vi "PathPlanner_Waypoint_New.vi"(9 "NextControl":T1={"X"=-9.9e+30, "Y"=-9.9e+30} {"Y" format="%14.3f"; "X" format="%14.3f"}, 10 "Anchor":T1 {"Y" format="%14.3f"; "X" format="%14.3f"}, 11 "PrevControl":T1={"X"=-9.9e+30, "Y"=-9.9e+30} {"Y" format="%14.3f"; "X" format="%14.3f"}) -> (3 "Waypoint":T2 {"nextControl"."Y" format="%14.3f"; "nextControl"."X" format="%14.3f"; "anchor"."Y" format="%14.3f"; "anchor"."X" format="%14.3f"; "prevControl"."Y" format="%14.3f"; "prevControl"."X" format="%14.3f"})   [LabVIEW 2019, in "PathPlanner24.lvlib"]
doc: "Convert bezier points to waypoints allowing them to be written to a JSON string.\n\nInputs: \n - Bezier - array of translation2s - List of bezier points\n\nOutputs:\n - waypoints - array of cluster - waypoints compatible with pathplanner path JSON strings."
uses:
  PathPlanner24.lvlib
  TypeDef/PathPlannerWaypoint.ctl
  <vilib>/Rock Robotics/WPI/ThirdParty/JAS_Junk/TrajLib/TypeDef/TRANSLATION2D.ctl
  <vilib>/Rock Robotics/WPI/ThirdParty/JAS_Junk/TrajLib/Trajectory_Library.lvlib
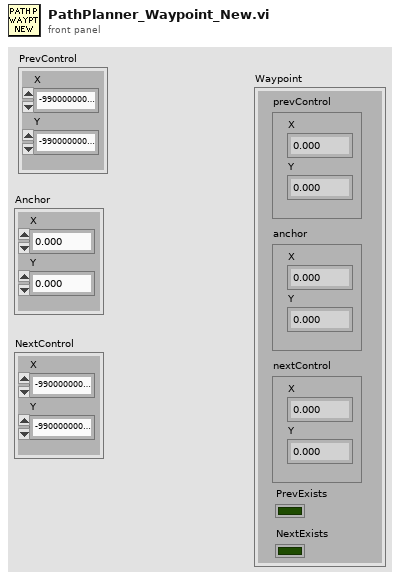
[diagram p1: front panel]
types:
  T1 = typedef "Trajectory_Library.lvlib/TRANSLATION2D.ctl" = cluster{"X":dbl, "Y":dbl}
  T2 = typedef "PathPlanner24.lvlib/PathPlannerWaypoint.ctl" = cluster{"prevControl":T1, "anchor":T1, "nextControl":T1, "PrevExists":bool, "NextExists":bool}
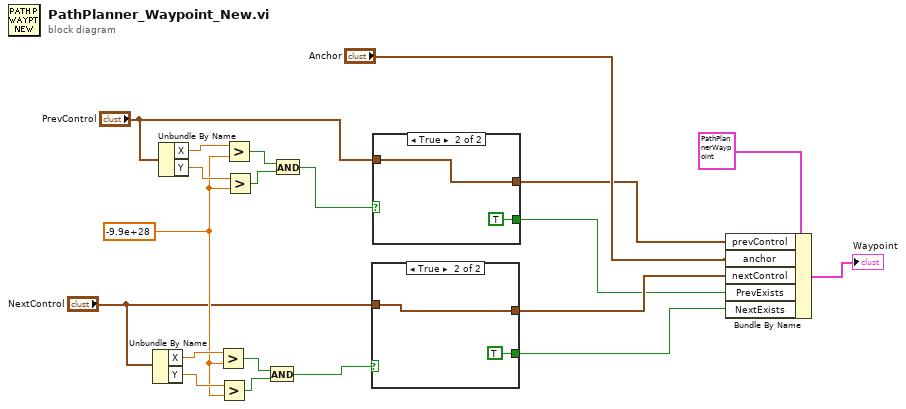
[diagram p0: block diagram]
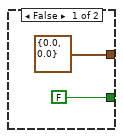
[diagram p2: hidden frame]
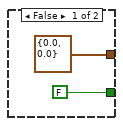
[diagram p3: hidden frame]
diagram:
  w4 = -9.9e+28
  n1 = Unbundle By Name("NextControl") -> ("X"=w8:dbl, "Y"=w7:dbl)
  n2 = Unbundle By Name("PrevControl") -> ("X"=w13:dbl, "Y"=w12:dbl)
  n3 = Greater?(x=w8, y=w4) -> (0:w5:bool)
  n4 = Greater?(x=w7, y=w4) -> (0:w6:bool)
  n5 = Greater?(x=w13, y=w4) -> (0:w10:bool)
  n6 = Greater?(x=w12, y=w4) -> (0:w11:bool)
  n7 = And(x=w5, y=w6) -> (x .and. y?=w3:bool)
  n8 = And(x=w10, y=w11) -> (x .and. y?=w9:bool)
  n9 = case shown="True" w3 {
    tunnel: [T1 {"X"=0.0, "Y"=0.0} ("prevControl") w24] -> w16
    tunnel: [FALSE TRUE] -> w14
    tunnel: "NextControl" -> [_ w24]
    frame False {
    }
    frame True {
    }
  }
  n10 = case shown="True" w9 {
    tunnel: [T1 {"X"=0.0, "Y"=0.0} ("prevControl") w28] -> w17
    tunnel: [FALSE TRUE] -> w15
    tunnel: "PrevControl" -> [_ w28]
    frame False {
    }
    frame True {
    }
  }
  n11 = Bundle By Name(cluster=T2 {"prevControl"={"X"=0.0, "Y"=0.0}, "anchor"={"X"=0.0, "Y"=0.0}, "nextControl"={"X"=0.0, "Y"=0.0}, "PrevExists"=FALSE, "NextExists"=FALSE} ("Waypoint"), "prevControl"=w17, "anchor"="Anchor", "nextControl"=w16, "PrevExists"=w15, "NextExists"=w14) -> (→"Waypoint":T2)
